vi "UserFile.vi"(8 "错误输入":errorcluster caption="错误输入（无错误）", 10 "UserPath in":path, 11 "Step":enum16{"Initial", "Write", "Read"}(ring)) -> (0 "错误输出":errorcluster, 3 "UserPath out":path)   [LabVIEW 2017]
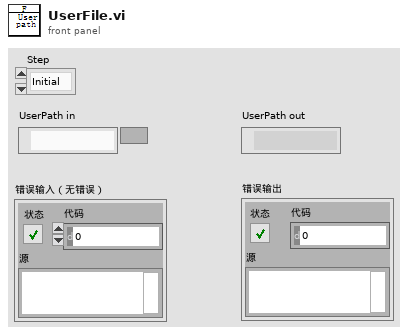
[diagram p1: front panel]
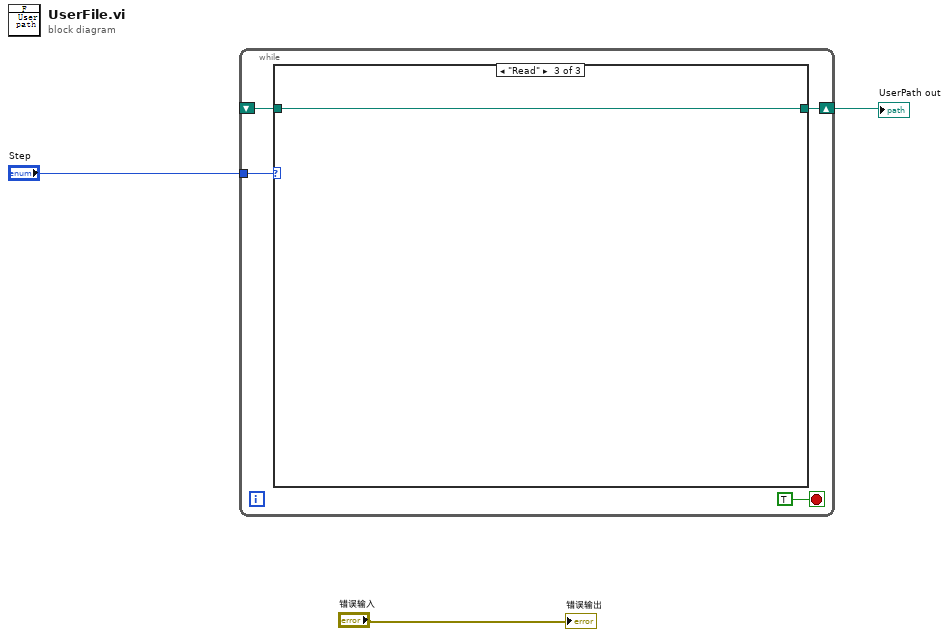
[diagram p0: block diagram]
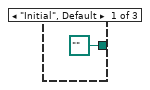
[diagram p2: hidden frame]
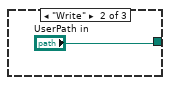
[diagram p3: hidden frame]
diagram:
  n1 = while {
    tunnel: "Step" -> [w6]
    shift-right: [w5] -> w1
    shift-left: _ -> [w4]
    stop <- TRUE stop-if-true
    n2 = case shown="\"Read\"" w6 {
      tunnel: [path "" ("MainPath in") "UserPath in" w10] -> w5
      tunnel: w4 -> [_ _ w10]
      frame "Initial", Default {
      }
      frame "Write" {
      }
      frame "Read" {
      }
    }
  }
  "UserPath out" <- w1
  "错误输出" <- "错误输入"
